vi "随机生成.vi"(9 "类型":enum16{"空白", "蛇", "食物", "墙", "传送门"}(ring)=enum."食物", 10 "上限":dbl, 11 "地图":u32[][](array[colorbox])) -> (3 "地图 2":u32[][](array[colorbox]))   [LabVIEW 2012]
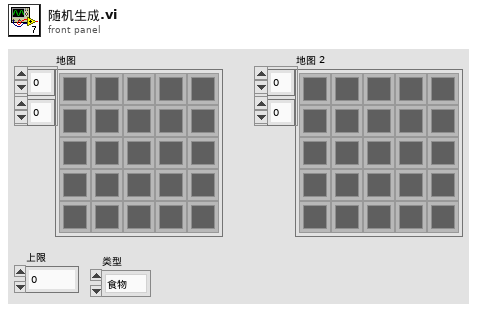
[diagram p1: front panel]
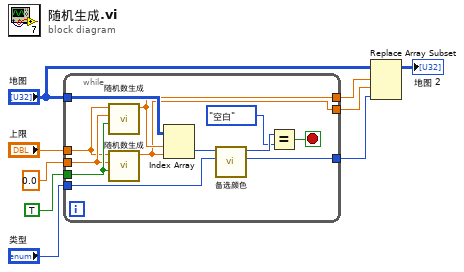
[diagram p0: block diagram]
diagram:
  n1 = while {
    tunnel: TRUE ("整数/浮点") -> [w21]
    tunnel: 0.0 ("下限") -> [w20]
    tunnel: "上限" -> [w19]
    tunnel: "地图" -> [w17]
    tunnel: [w13] -> w3
    tunnel: [w12] -> w5
    tunnel: [w11] -> w4
    tunnel: "类型" -> [w10]
    stop <- w18 stop-if-true
    n2 = call "随机数生成.vi"("整数/浮点"=w21, "下限"=w20, "上限"=w19) -> ("输出"=w12:dbl)  [unwired: 8 in]
    n3 = call "随机数生成.vi"("整数/浮点"=w21, "下限"=w20, "上限"=w19) -> ("输出"=w11:dbl)  [unwired: 8 in]
    n4 = Index Array(array=w17, index (row)=w12, index (col)=w11) -> (element=w16:u32)
    n5 = call "备选颜色.vi"("索引2"=w10, "颜色1"=w16) -> ("颜色2"=w13:u32, "索引1"=w15:enum16{"空白", "蛇", "食物", "墙", "传送门"})  [unwired: 8 in]
    n6 = Equal?(x=w15, y=enum16{"空白", "蛇", "食物", "墙", "传送门"}."空白") -> (x = y?=w18:bool)
  }
  n7 = Replace Array Subset(array="地图", new element=w3, index (row)=w5, index (col)=w4) -> (→"地图 2":u32[][])
